vi "_AttributeDataReady.vi"() -> (0 "attribute data ready":T1)   [LabVIEW 2014, in "tango.lvlib"]
uses:
  tango.lvlib
  Private VIs/Events/_AttributeDataReady_t.ctl
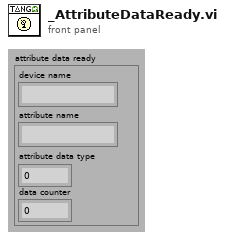
[diagram p1: front panel]
types:
  T1 = typedef "tango.lvlib/_AttributeDataReady_t.ctl" = cluster{"device name":string, "attribute name":string, "attribute data type":i16, "data counter":i16}
  T2 = cluster{"device name":string, "attribute name":string, "attribute data type":i32, "data counter":i32}
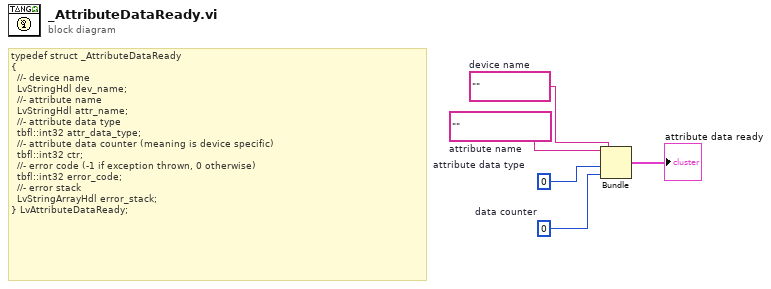
[diagram p0: block diagram]
diagram:
  w2 = ""  # device name
  w3 = ""  # attribute name
  w4 = 0  # data counter
  w5 = 0  # attribute data type
  # "typedef struct _AttributeDataReady\n{\n  //- device name\n  LvStringHdl dev_name;\n  //- attribute name\n  LvStringHdl attr_name;\n  //- attribute data type\n  tbfl::int32 attr_data_type;\n  //- attribute data counter (meaning is device specific)\n  tbfl::int32 ctr;\n  //- error code (-1 if exception thrown, 0 otherwise)\n  tbfl::int32 error_code;\n  //- error stack\n  LvStringArrayHdl error_stack;\n} LvAttributeDataReady;"
  n1 = Bundle("device name"=w2, "attribute name"=w3, "attribute data type"=w5, "data counter"=w4) -> (→"attribute data ready":T2)  [unwired: 1 in]
